vi "TimedLog.vi"(8 "error in (no error)":errorcluster, 10 "Message":string, 11 "Logger in":refnum<class "Logger.lvclass">) -> (0 "error out":errorcluster, 2 "logged string":string, 3 "Logger out":refnum<class "Logger.lvclass">)   [LabVIEW 2011, in "Logger.lvclass"]
doc: "logs a message to the standard message log, along with a timestamp."
uses:
  Logger.lvclass
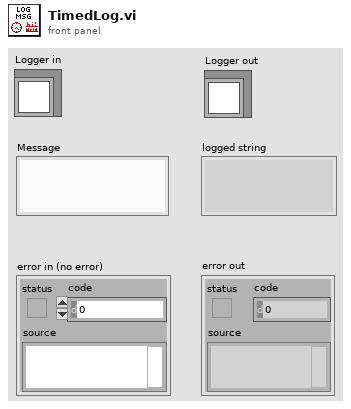
[diagram p1: front panel]
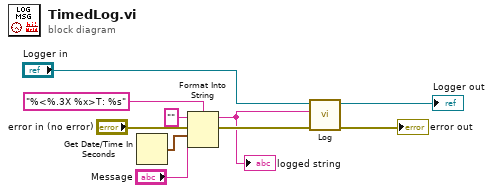
[diagram p0: block diagram]
diagram:
  n1 = Get Date/Time In Seconds() -> (seconds since 1Jan1904=w5:timestamp)
  n2 = Format Into String(format string="%<%.3X %x>T: %s" ("initial string"), initial string="", error in="error in (no error)", w5, "Message") -> (resulting string=w6:string, error out=w7:errorcluster)
  "logged string" <- w6
  n3 = call "Log.vi"("error in (no error)"=w7, "Message"=w6, "Logger in"="Logger in") -> ("error out"=→"error out":errorcluster, "Logger out"=→"Logger out":refnum<class "Logger.lvclass">)  [unwired: 7 in]
